vi "Start Stop Datalog.vi"(8 "error in (no error)":errorcluster, 10 "Datalog File Name":string="\"0\"", 11 "VISA resource name":refnum<visa-resource-name>) -> (0 "error out":errorcluster, 3 "VISA resource name out":refnum<visa-resource-name>)   [LabVIEW 2010, in "Temptronic TP04300.lvlib"]
doc: "This VI turns the datalogging On or Off, depending on the Datalog File Name value.\n\n Use Command Argument \n = 0 to turn the datalogging off\n = <file_name> to turn the datalogging on\n\nNote: The file name or 0 should be in quotes.\n\nNote: If the file already exists, it will automatically be overwritten."
uses:
  Temptronic TP04300.lvlib
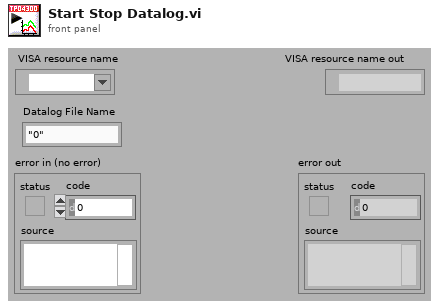
[diagram p1: front panel]
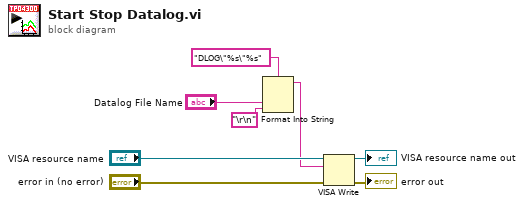
[diagram p0: block diagram]
diagram:
  n1 = Format Into String(format string="DLOG\"%s\"%s" ("multi-line string"), "Datalog File Name", "\r\n") -> (resulting string=w3:string)  [unwired: 2 in, 1 out]
  n2 = VISA Write(VISA resource name="VISA resource name", write buffer=w3, error in (no error)="error in (no error)") -> (VISA resource name out=→"VISA resource name out":refnum<visa-resource-name>, error out=→"error out":errorcluster)  [unwired: 1 out]
